vi "IPC-ModbusSerial-WriteMulRegisters.vi"(5 "parity (Even)":u16(ring)=2 caption="奇偶（偶）" items=["无", "奇", "偶"], 6 "baud rate (9600)":u32=9600 caption="波特率(9600)", 7 "VISA resource name":refnum<visa-resource-name>="COM1" caption="VISA资源名称", 8 "error in (no error)":errorcluster caption="错误输入（无错误）", 9 "holding register values":u16[](array[numeric]) caption="保持寄存器值", 10 "starting address":u16 caption="起始地址", 11 "unit ID":u8=1 caption="单元ID") -> (0 "error out":errorcluster caption="错误输出")   [LabVIEW 2014]
uses:
  <vilib>/Modbus/master/Create Master Instance (Serial).vi
  <vilib>/Modbus/master/Modbus Master.lvclass
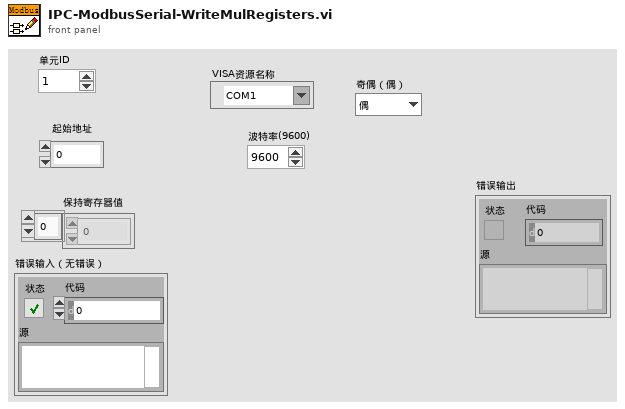
[diagram p1: front panel]
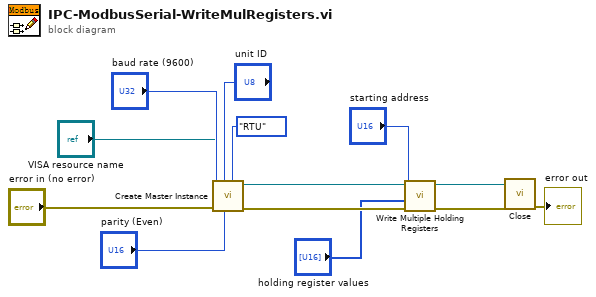
[diagram p0: block diagram]
diagram:
  n1 = call-poly <vilib>:"Create Master Instance.vi"("serial type"=enum16{"RTU", "ASCII"}."RTU", "parity (Even)"="parity (Even)", "unit ID"="unit ID", "error in (no error)"="error in (no error)", "baud rate (9600)"="baud rate (9600)", "VISA resource name"="VISA resource name") -> ("error out"=w7:errorcluster, "serial master instance"=w8:refnum<class "Modbus Master.lvclass">)  [unwired: 4 in]
  n2 = call-dynamic "Write Multiple Holding Registers.vi"("error in (no error)"=w7, "holding register values"="holding register values", "starting address"="starting address", "Modbus master in"=w8) -> ("error out"=w6:errorcluster, "Modbus master out"=w5:refnum<class "Modbus Master.lvclass">)  [unwired: 6 in]
  n3 = call-dynamic "Close.vi"("error in (no error)"=w6, "Modbus master in"=w5) -> ("error out"=→"error out":errorcluster)  [unwired: 9 in]
